vi "Motion Done.vi"(8 "error in (no error)":errorcluster, 10 "Axis":i32, 11 ".NET Refnum in":refnum<k24>) -> (0 "error out":errorcluster, 3 "Done":bool)   [LabVIEW 2019]
uses:
  Newport.ESP301.CommandInterface
  ESP301.lvlib
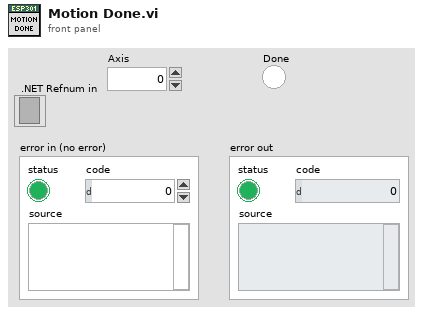
[diagram p1: front panel]
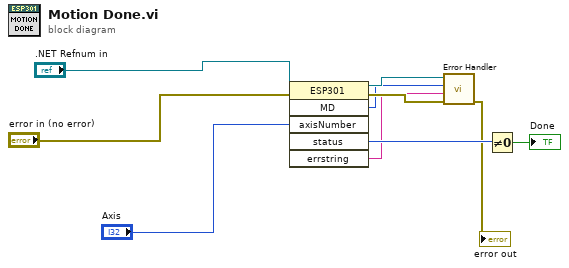
[diagram p0: block diagram]
diagram:
  n1 = invoke class="ESP301" method="MD"(reference=".NET Refnum in", error in="error in (no error)", "axisNumber"="Axis") -> (reference out=w3:refnum<k24>, error out=w9:errorcluster, "MD"=w2:i32, "status"=w6:i32, "errstring"=w1:string)  [unwired: 3 in, 1 out]
  n2 = call "Error Handler.vi"("error in (no error)"=w9, "value"=w1, "OpenInstrument"=w2, ".NET Refnum in"=w3) -> ("error out"=→"error out":errorcluster)  [unwired: 6 in, 1 out]
  n3 = Not Equal To 0?(x=w6) -> (x != 0?=→"Done":bool)
